vi "create.OrderExecuted.vi"(11 "OrderExecuted.Parameters":T1={"Time Offset"=447000, "Order Id"="ORID0001", "Executed Quantity"=20000, "Execution Id"="AAPL"}) -> (2 "Bytes.Out":u8[](array[numeric]) format="%.0x", 3 "MessageBase out":refnum<class "OrderExecuted.lvclass">)   [LabVIEW 2020]
uses:
  OrderExecuted/OrderExecuted.Parameters.ctl
  OrderExecuted/OrderExecuted.lvclass
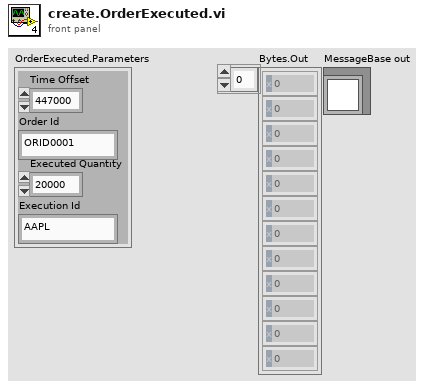
[diagram p1: front panel]
types:
  T1 = typedef "OrderExecuted.lvclass/OrderExecuted.Parameters.ctl" = cluster{"Time Offset":u32, "Order Id":string, "Executed Quantity":u32, "Execution Id":string}
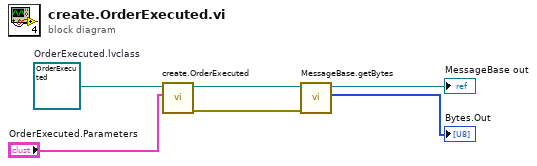
[diagram p0: block diagram]
diagram:
  w3 = refnum<class "OrderExecuted.lvclass"> refnum  # OrderExecuted.lvclass
  n1 = call-dynamic "create.OrderExecuted.vi"("OrderExecuted.Parameters"="OrderExecuted.Parameters", "OrderExecuted in"=w3) -> ("error out"=w5:errorcluster, "OrderExecuted out"=w4:refnum<class "OrderExecuted.lvclass">)  [unwired: 8 in]
  n2 = call-dynamic "MessageBase.getBytes.vi"("error in (no error)"=w5, "MessageBase in"=w4) -> ("Bytes.out"=→"Bytes.Out":u8[], "MessageBase out"=→"MessageBase out":refnum<class "OrderExecuted.lvclass">)  [unwired: 7 in, 1 out]
